vi "Test3.vi"() -> ()   [LabVIEW 2013]
panel:
  out "*(type *) &x":string
  out "spreadsheet string":string
  out "subarray":string[](array[string])
  out "size(s)":i32
  out "hex integer string":string[](array[string])
  out "String":string
  out "data":string
  in  "byte order (0:big-endian, network order)":T1(ring)
  in  "error in":errorcluster
  out "error out":errorcluster
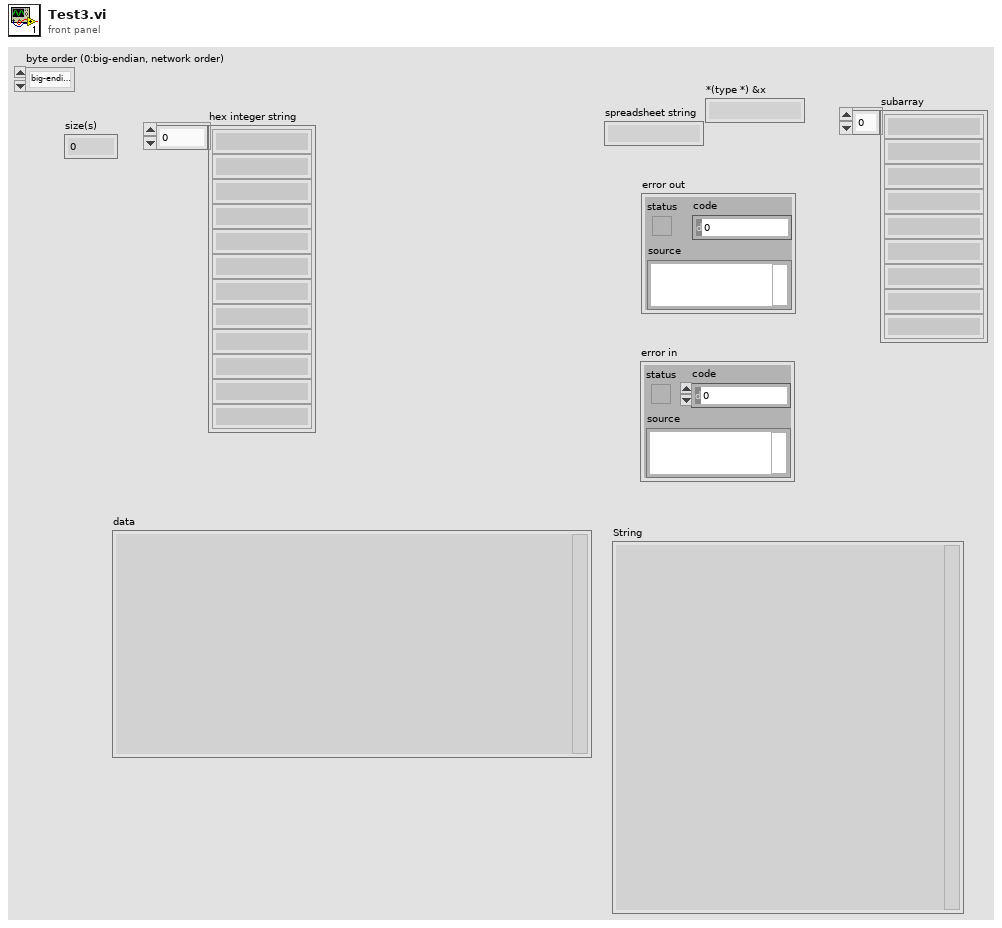
[diagram p1: front panel]
types:
  T1 = enum16{"big-endian, network order", "native, host order", "little-endian"}
  T2 = enum16{"open", "replace", "create", "open or create", "replace or create", "replace or create with confirmation"}
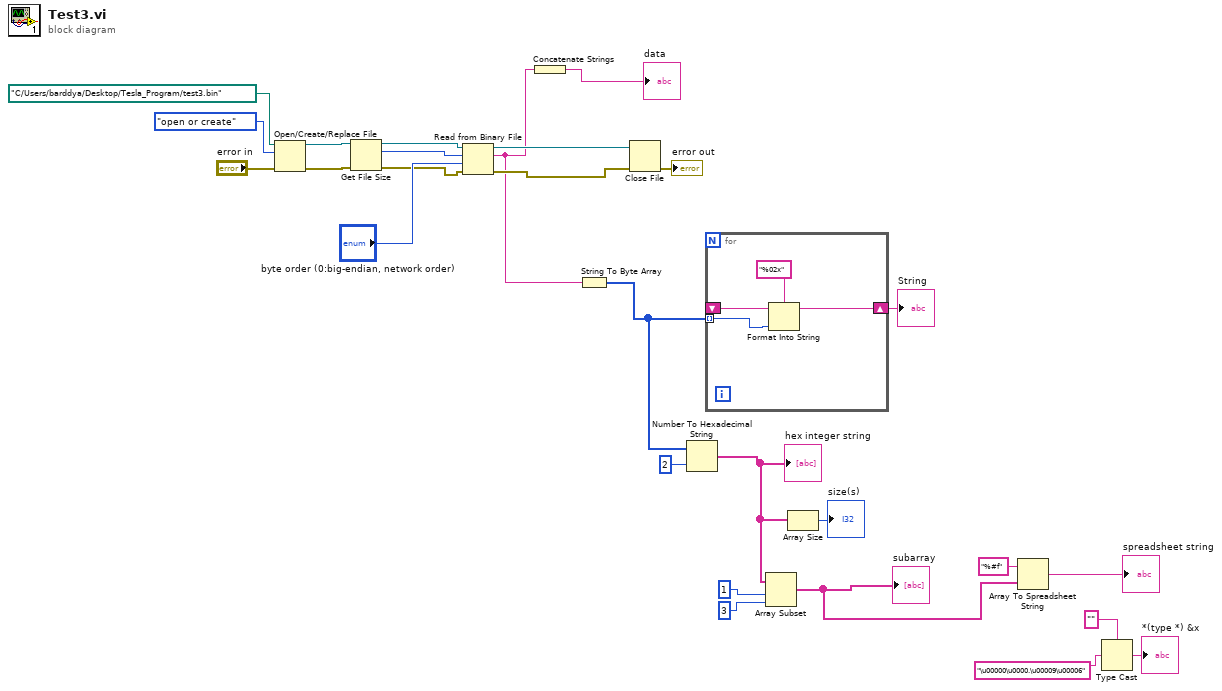
[diagram p0: block diagram]
diagram:
  n1 = Open/Create/Replace File(file path (use dialog)=path "C:/Users/barddya/Desktop/Tesla_Program/test3.bin", error in="error in", operation (0:open)=T2."open or create") -> (refnum out=w20:refnum<file>, error out=w18:errorcluster)  [unwired: 3 in, 1 out]
  n2 = Get File Size(file=w20, error in=w18) -> (refnum out=w19:refnum<file>, size (in bytes)=w16:i64, 0:w17:errorcluster)
  n3 = Read from Binary File(8:w17, 9:"byte order (0:big-endian, network order)", 10:w16, 11:w19) -> (0:w23:errorcluster, 2:w14:string, 3:w21:refnum<file>)  [unwired: 2 in, 1 out]
  n4 = Concatenate Strings(w14) -> (→"data":string)
  n5 = String To Byte Array(string=w14) -> (unsigned byte array=w12:u8[])
  n6 = Close File(refnum=w21, error in=w23) -> (error out=→"error out":errorcluster)  [unwired: 1 out]
  n7 = Number To Hexadecimal String(1:2, 2:w12) -> (0:w9:string[])
  "hex integer string" <- w9
  n8 = for {
    tunnel: w12 -> [w31] mode=indexing
    shift-right: [w30] -> w13
    shift-left: _ -> [w29]
    n9 = Format Into String(format string="%02x", initial string=w29, w31) -> (resulting string=w30:string)  [unwired: 1 in, 1 out]
  }
  "String" <- w13
  n10 = Array Subset(array=w9, index=1, length=3) -> (w6:string[])
  "subarray" <- w6
  n11 = Array Size(array=w9) -> (size(s)=→"size(s)":i32)
  n12 = Array To Spreadsheet String(array=w6, 3:"%#f" ("format string")) -> (spreadsheet string=→"spreadsheet string":string)  [unwired: 1 in]
  n13 = Type Cast(type="", x="\u00000\u0000.\u00009\u00006") -> (*(type *) &x=→"*(type *) &x":string)
